vi "UI Update Frame Image.vi"(8 "error in (no error)":errorcluster, 11 "LF2R IDE in":refnum<class "LF2R IDE.lvclass">) -> (0 "error out":errorcluster, 3 "LF2R IDE out":refnum<class "LF2R IDE.lvclass">)   [LabVIEW 2018, in "LF2R IDE.lvlib" / "LF2R IDE.lvclass"]
uses:
  LF2R IDE.lvclass
  LF2R IDE.lvclass/LF2R IDE.ctl
  Image/Image Process.lvclass
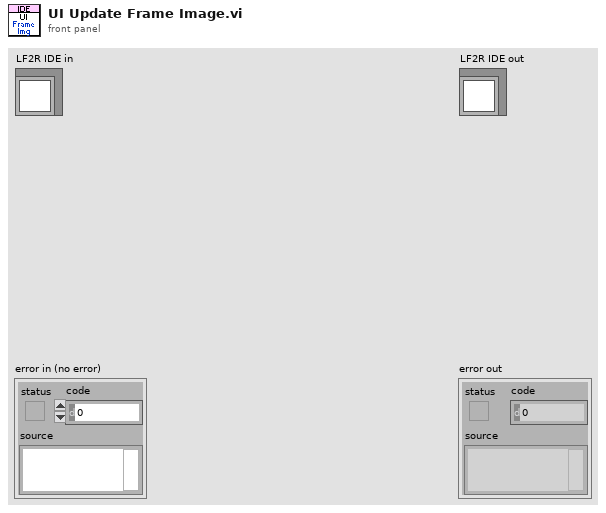
[diagram p1: front panel]
types:
  T1 = cluster{"left":i16, "top":i16, "right":i16, "bottom":i16}
  T2 = typedef "IMAQ Image.ctl" = refnum<image>
  T3 = typedef "imagedata.ctl" = cluster{"image type":i32, "image depth":i32, "image":u8[], "mask":u8[], "colors":u32[], "Rectangle":cluster{"left":i16, "top":i16, "right":i16, "bottom":i16}}
  T4 = typedef "Image Json Parser.lvclass/Img Json Data.ctl" = cluster{"frames":T5[], "meta":T6}
  T5 = typedef "Image Json Parser.lvclass/Img Json Frames.ctl" = cluster{"frame":cluster{"x":i32, "y":i32, "w":i32, "h":i32}, "rotated":bool, "trimmed":bool, "spriteSourceSize":cluster{"x":i32, "y":i32, "w":i32, "h":i32}, "sourceSize":cluster{"w":i32, "h":i32}}
  T6 = typedef "Image Json Parser.lvclass/Img Json Meta.ctl" = cluster{"app":string, "version":string, "image":string, "format":string, "size":cluster{"w":i32, "h":i32}, "scale":string}
  T7 = typedef "Image Type" = u32
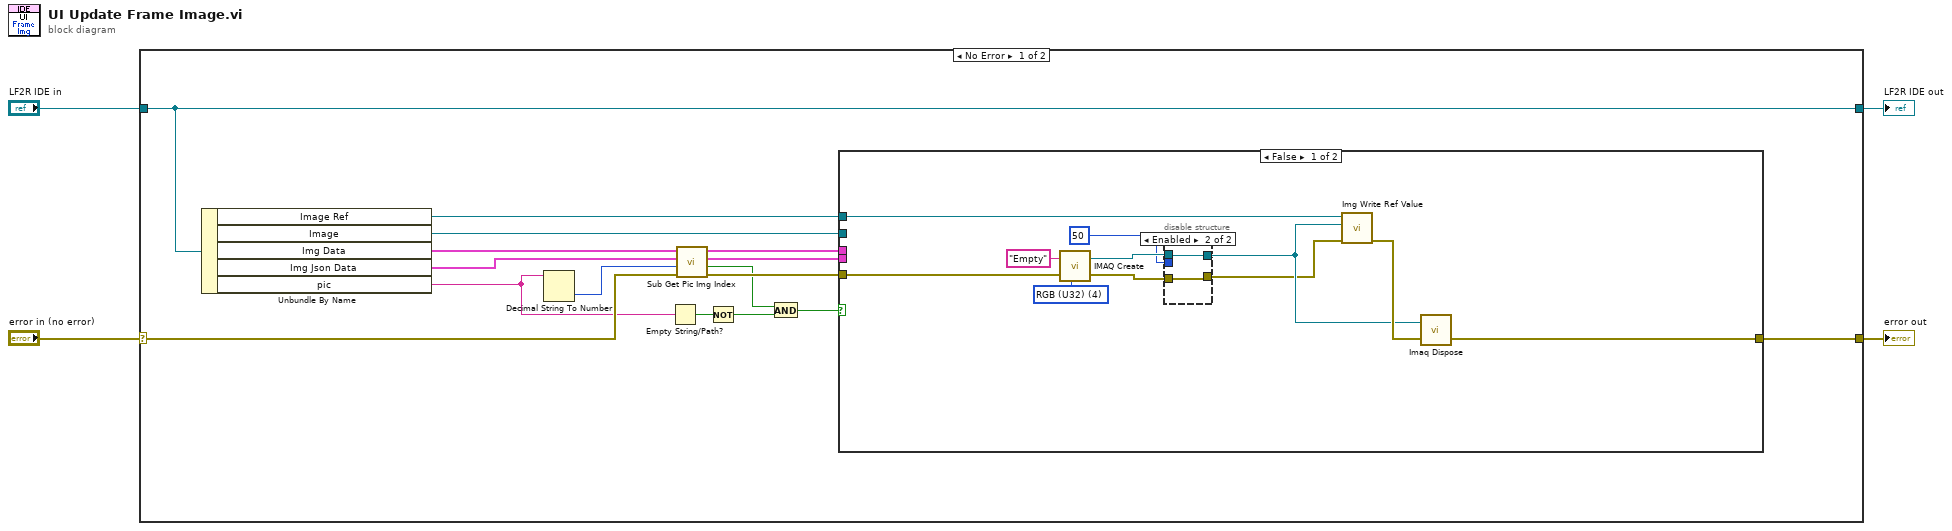
[diagram p0: block diagram]
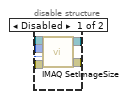
[diagram p2: hidden frame]
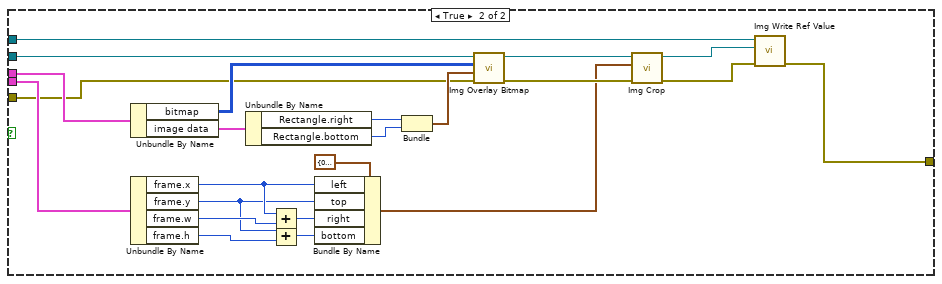
[diagram p3: hidden frame]
diagram:
  n1 = case shown="No Error" "error in (no error)" {
    selector: "error in (no error)" -> [w18 w63]
    tunnel: [w12 w63] -> w3
    tunnel: [w11 w62] -> w1
    tunnel: "LF2R IDE in" -> [w11 w62]
    frame No Error {
      n2 = Unbundle By Name(w11) -> ("Image Ref"=w13:refnum<vi>, "Image"=w16:T2, "Img Data"=w20:cluster{"image data":T3, "bitmap":u32[][]}[], "Img Json Data"=w19:T4[], "pic"=w9:string)
      n3 = Decimal String To Number(string=w9) -> (number=w10:i32)  [unwired: 2 in, 1 out]
      n4 = Empty String/Path?(string/path=w9) -> (empty?=w8:bool)
      n5 = call "Sub Get Pic Img Index.vi"("error in (no error)"=w18, "Pic Num"=w10, "Img Json Data"=w19, "Img Data"=w20) -> ("error out"=w14:errorcluster, "Found?"=w6:bool, "frames"=w17:T5, "Img Data indexed"=w15:cluster{"image data":T3, "bitmap":u32[][]})  [unwired: 4 in]
      n6 = Not(x=w8) -> (.not. x?=w7:bool)
      n7 = And(x=w6, y=w7) -> (x .and. y?=w5:bool)
      n8 = case shown="False" w5 {
        tunnel: w17 -> [_ w54]
        tunnel: w16 -> [_ w51]
        tunnel: w15 -> [_ w50]
        tunnel: w14 -> [w29 w44]
        tunnel: w13 -> [w31 w42]
        tunnel: [w27 w39] -> w12
        frame False {
          w28 = T7 4 items=["Grayscale (U8)", "Grayscale (I16)", "Grayscale (SGL)", "Complex (CSG)", "RGB (U32)", "HSL (U32)", "RGB (U64)", "Grayscale (U16)"] ("Image Type")
          n9 = call "IMAQ Create"("Image Name"="Empty", "Image Type"=w28, "error in (no error)"=w29) -> ("New Image"=w25:T2, "error out"=w23:errorcluster)  [unwired: 2 in]
          n10 = disable-structure shown="Enabled" {
            disable-tunnel: w25 -> [w36 w37]
            disable-tunnel: [w35 w37] -> w24
            disable-tunnel: w23 -> [w34 w38]
            disable-tunnel: [w33 w38] -> w22
            disable-tunnel: 50 ("X Resolution") -> [w32 _]
            frame Disabled {
              n11 = call "IMAQ SetImageSize"("error in (no error)"=w34, "Y Resolution"=w32, "X Resolution"=w32, "Image"=w36) -> ("error out"=w33:errorcluster, "Image Out"=w35:T2)  [unwired: 1 in]
            }
            frame Enabled {
            }
          }
          n12 = call "Img Write Ref Value.vi"("error in (no error)"=w22, "Image"=w24, "Image Ref"=w31) -> ("error out"=w26:errorcluster)  [unwired: 8 in]
          n13 = call "Imaq Dispose"("Image"=w24, "error in (no error)"=w26) -> ("error out"=w27:errorcluster)  [unwired: 4 in]
        }
        frame True {
          n14 = Unbundle By Name(w50) -> ("bitmap"=w49:u32[][], "image data"=w46:T3)
          n15 = Unbundle By Name(w54) -> ("frame.x"=w60:i32, "frame.y"=w57:i32, "frame.w"=w59:i32, "frame.h"=w55:i32)
          n16 = Unbundle By Name(w46) -> ("Rectangle.right"=w48:i16, "Rectangle.bottom"=w47:i16)
          n17 = Add(x=w60, y=w59) -> (x+y=w58:i32)
          n18 = Add(x=w57, y=w55) -> (x+y=w56:i32)
          n19 = Bundle By Name(cluster=T1 {"left"=0, "top"=0, "right"=269, "bottom"=269} ("Rectangle"), "left"=w60, "top"=w57, "right"=w58, "bottom"=w56) -> (w43:T1)
          n20 = Bundle("right"=w48, "bottom"=w47) -> (w45:cluster{"right":i16, "bottom":i16})  [unwired: 1 in]
          n21 = call "Img Overlay Bitmap.vi"("error in (no error)"=w44, "Size"=w45, "Bitmap"=w49, "Image"=w51) -> ("error out"=w52:errorcluster, "Image Out"=w53:T2)  [unwired: 6 in]
          n22 = call "Img Crop.vi"("error in (no error)"=w52, "Rectangle"=w43, "Image Src"=w53) -> ("error out"=w40:errorcluster, "Image Out"=w41:T2)  [unwired: 7 in]
          n23 = call "Img Write Ref Value.vi"("error in (no error)"=w40, "Image"=w41, "Image Ref"=w42) -> ("error out"=w39:errorcluster)  [unwired: 8 in]
        }
      }
    }
    frame Error {
    }
  }
  "error out" <- w3
  "LF2R IDE out" <- w1
